vi "DAQ.DAQmx Asynch Write.vi"(0 "Refnum in":refnum<k21>, 1 "auto start":bool, 7 "data":waveform(dbl)[](array[waveform]), 9 "timeout":dbl, 11 "error in (no error)":errorcluster, 12 "ID in":i32) -> (4 "Refnum out":refnum<k21>, 10 "number of samples written per channel":u32, 14 "ID out":i32, 15 "error out":errorcluster)   [LabVIEW 2019, in "Instrument.Lockin.lvlib" / "Instrument.DAQ.lvclass"]
uses:
  Instrument.DAQ.lvclass
  <vilib>/DAQmx/write.llb/DAQmx Write (Analog 1D Wfm NChan NSamp).vi
  <vilib>/DAQmx/miscellaneous.llb/DAQmx Fill In Error Info.vi
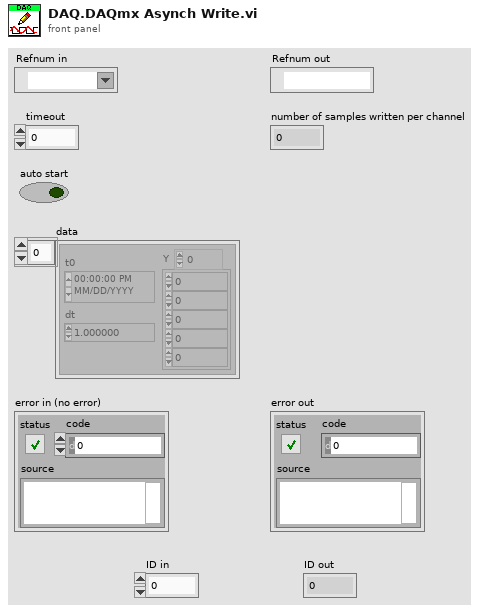
[diagram p1: front panel]
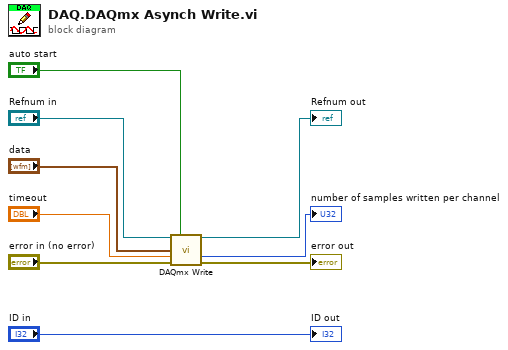
[diagram p0: block diagram]
diagram:
  n1 = call-poly <vilib>:"DAQmx Write.vi"("task/channels in"="Refnum in", "auto start"="auto start", "data"="data", "timeout"="timeout", "error in"="error in (no error)") -> ("task out"=→"Refnum out":refnum<k21>, "number of samples written per channel"=→"number of samples written per channel":u32, "error out"=→"error out":errorcluster)  [unwired: 8 in]
  "ID out" <- "ID in"
